vi "DistToNearestEnd.vi"(8 "Any End":dbl, 9 "Z":dbl, 10 "X":dbl, 11 "All Lines 2":T1) -> (1 "Index":i32, 2 "Distance to nearest end":dbl, 3 "In range?":bool)   [LabVIEW 2014]
uses:
  Libraries/Map Data Folder/All-Lines.ctl
  Libraries/Map Data Folder/LineCluster.ctl
  Libraries/Map Data Folder/LineConnection.ctl
  Libraries/Map Data Folder/Map Data.lvlib
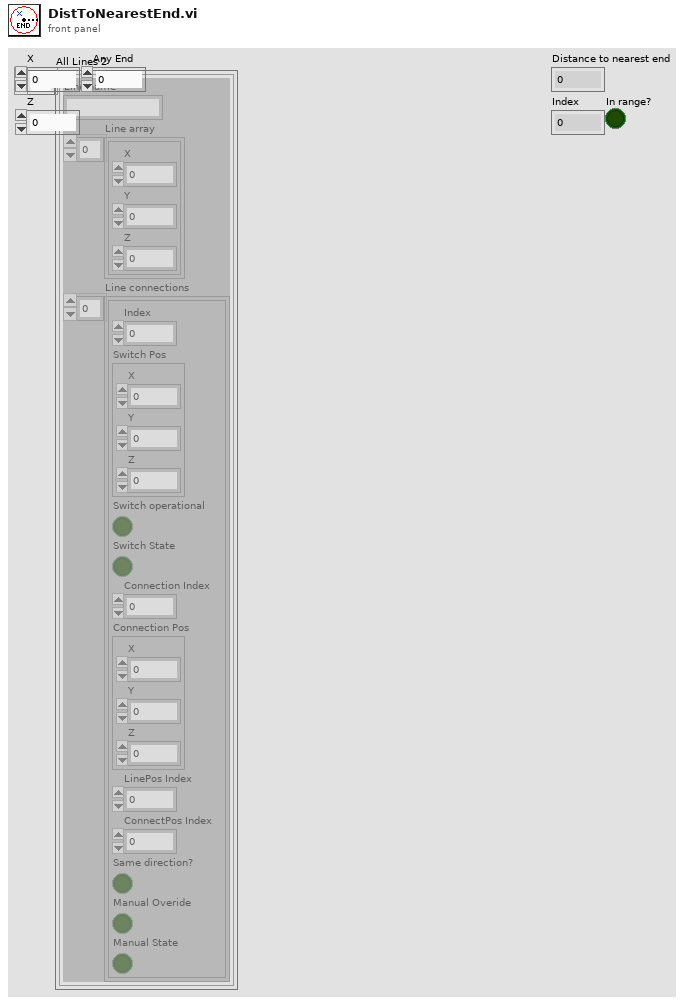
[diagram p1: front panel]
types:
  T1 = typedef "Map Data.lvlib/All-Lines.ctl" = T2[]
  T2 = typedef "Map Data.lvlib/LineCluster.ctl" = cluster{"Line name":string, "Line array":cluster{"X":dbl, "Y":dbl, "Z":dbl}[], "Line connections":T3[]}
  T3 = typedef "LineConnection.ctl" = cluster{"Index":i32, "Switch Pos":cluster{"X":dbl, "Y":dbl, "Z":dbl}, "Switch operational":bool, "Switch State":bool, "Connection Index":i32, "Connection Pos":cluster{"X":dbl, "Y":dbl, "Z":dbl}, "LinePos Index":i32, "ConnectPos Index":i32, "Same direction?":bool, "Manual Overide":bool, "Manual State":bool}
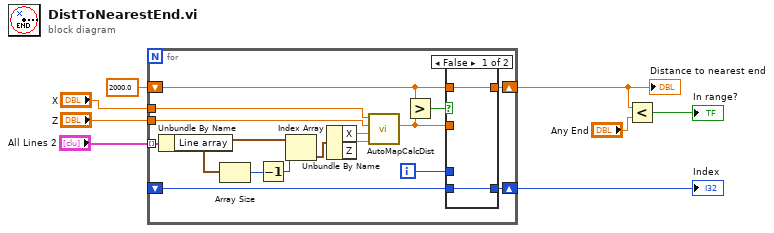
[diagram p0: block diagram]
diagram:
  n1 = for {
    tunnel: "All Lines 2" -> [w24] mode=indexing
    tunnel: "Z" -> [w23]
    tunnel: "X" -> [w22]
    shift-right: [w13] -> w3
    shift-left: 2000.0 ("Distance") -> [w12]
    shift-right: [w11] -> w4
    shift-left: _ -> [w9]
    i -> [w10]
    n2 = Unbundle By Name(w24) -> ("Line array"=w17:cluster{"X":dbl, "Y":dbl, "Z":dbl}[])
    n3 = Array Size(array=w17) -> (size(s)=w18:i32)
    n4 = Decrement(x=w18) -> (x-1=w16:i32)
    n5 = Index Array(array=w17, index=w16) -> (element=w19:cluster{"X":dbl, "Y":dbl, "Z":dbl})
    n6 = Unbundle By Name(w19) -> ("X"=w21:dbl, "Z"=w20:dbl)
    n7 = call "AutoMapCalcDist.vi"("Y2"=w20, "X2"=w21, "Y1"=w23, "X1"=w22) -> ("Distance"=w14:dbl)  [unwired: 7 in]
    n8 = Greater?(x=w12, y=w14) -> (0:w15:bool)
    n9 = case shown="False" w15 {
      tunnel: w14 -> [_ w28]
      tunnel: [w26 w28] -> w13
      tunnel: w12 -> [w26 _]
      tunnel: w9 -> [w25 _]
      tunnel: [w25 w27] -> w11
      tunnel: w10 -> [_ w27]
      frame False {
      }
      frame True {
      }
    }
  }
  "Distance to nearest end" <- w3
  "Index" <- w4
  n10 = Less?(x=w3, y="Any End") -> (x < y?=→"In range?":bool)
